vi "QueryAxisParameter(Int).vi"(7 "Cmd":string, 8 "error in (no error)":errorcluster, 11 "Picomoto8742ControllerClass in":refnum<class "Picomoto8742ControllerClass.lvclass">) -> (0 "error out":errorcluster, 2 "ValueOut":i32, 3 "Picomoto8742ControllerClass Out":refnum<class "Picomoto8742ControllerClass.lvclass">)   [LabVIEW 2013, in "Picomoto8742ControllerClass.lvclass"]
doc: "Query a numeric parameter (Int32) from the physical device"
uses:
  Picomoto8742ControllerClass.lvclass
  Picomoto8742ControllerClass.lvclass/Picomoto8742ControllerClass.ctl
  PicoMotor8472Comm/PicoMotor8742Comm.lvclass
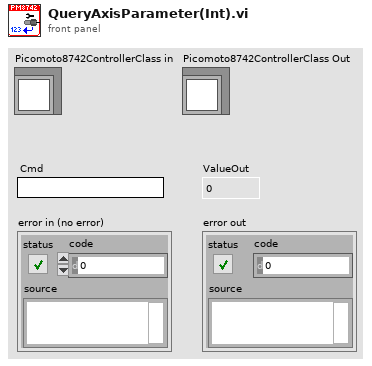
[diagram p1: front panel]
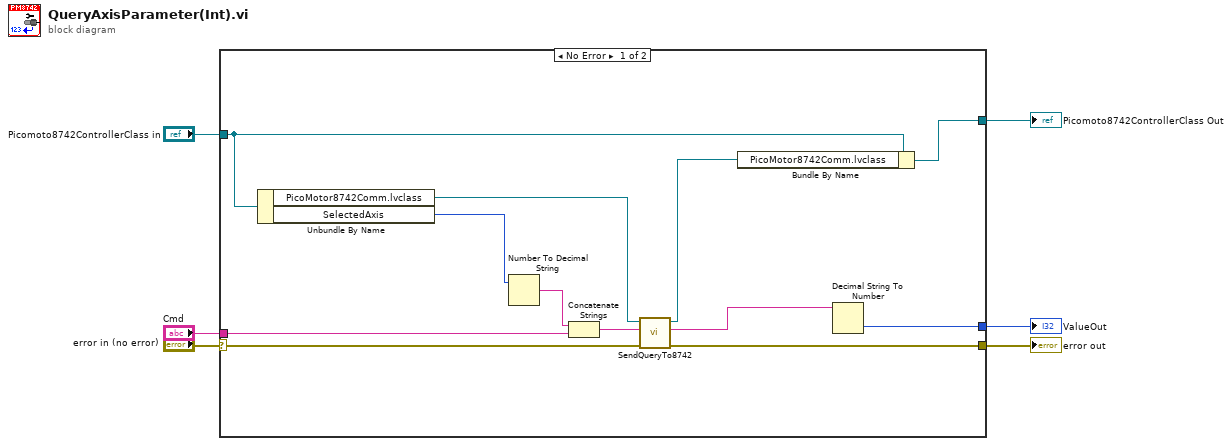
[diagram p0: block diagram]
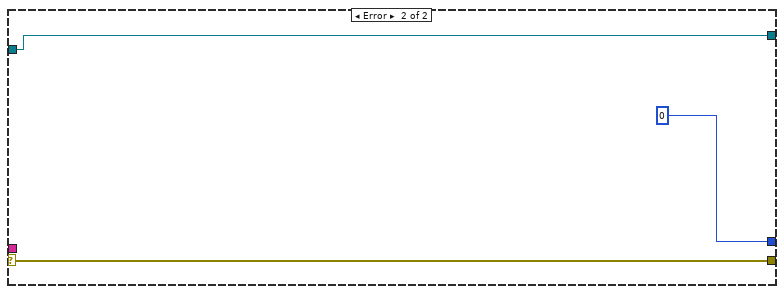
[diagram p2: hidden frame]
diagram:
  n1 = case shown="No Error" "error in (no error)" {
    selector: "error in (no error)" -> [w15 w21]
    tunnel: "Cmd" -> [w8 _]
    tunnel: [w14 w21] -> w5
    tunnel: [w18 0] -> w4
    tunnel: "Picomoto8742ControllerClass in" -> [w13 w19]
    tunnel: [w12 w19] -> w1
    frame No Error {
      n2 = Unbundle By Name(w13) -> ("PicoMotor8742Comm.lvclass"=w17:refnum<class "PicoMotor8742Comm.lvclass">, "SelectedAxis"=w10:u32)
      n3 = Number To Decimal String(number=w10) -> (decimal integer string=w9:string)  [unwired: 1 in]
      n4 = Concatenate Strings(w9, w8) -> (w7:string)
      n5 = call-dynamic "SendQueryTo8742.vi"("error in (no error)"=w15, "Command"=w7, "PicoMotor8742Comm in"=w17) -> ("error out"=w14:errorcluster, "Reply"=w16:string, "PicoMotor8742Comm out"=w11:refnum<class "PicoMotor8742Comm.lvclass">)  [unwired: 6 in]
      n6 = Bundle By Name(cluster=w13, "PicoMotor8742Comm.lvclass"=w11) -> (w12:refnum<class "Picomoto8742ControllerClass.lvclass">)
      n7 = Decimal String To Number(string=w16) -> (number=w18:i32)  [unwired: 2 in, 1 out]
    }
    frame Error {
    }
  }
  "error out" <- w5
  "ValueOut" <- w4
  "Picomoto8742ControllerClass Out" <- w1
